vi "Read PRAGMA key Command.vi"(8 "error in (no error)":errorcluster, 11 "SQLite in":refnum<class "SQLite.lvclass">) -> (0 "error out":errorcluster, 2 "PRAGMA key Command":string, 3 "SQLite out":refnum<class "SQLite.lvclass">)   [LabVIEW 2021, in "SQLite.lvclass"]
uses:
  SQLite.lvclass
  SQLite.lvclass/SQLite.ctl
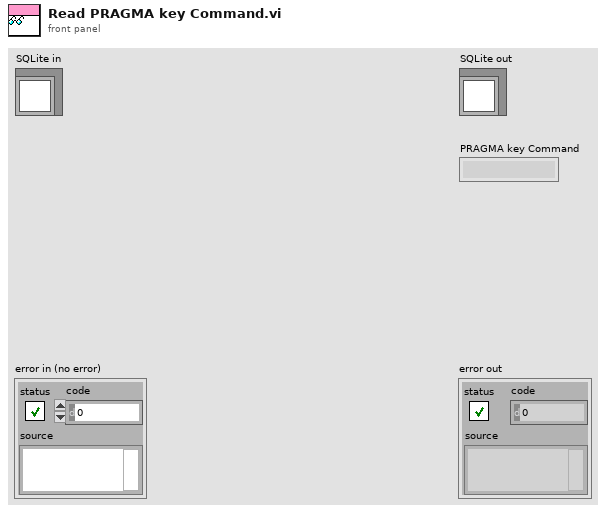
[diagram p1: front panel]
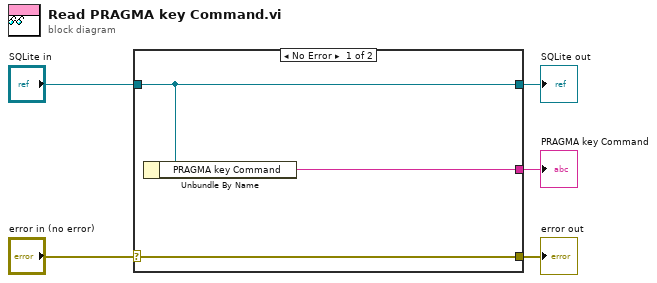
[diagram p0: block diagram]
diagram:
  n1 = case shown="No Error" "error in (no error)" {
    selector: "error in (no error)" -> [w8 w9]
    tunnel: [w8 w9] -> w4
    tunnel: [w7 w10] -> w2
    tunnel: "SQLite in" -> [w7 w10]
    tunnel: [w6 _] -> w1
    frame No Error {
      n2 = Unbundle By Name(w7) -> ("PRAGMA key Command"=w6:string)
    }
    frame Error {
    }
  }
  "error out" <- w4
  "SQLite out" <- w2
  "PRAGMA key Command" <- w1
